vi "CTRE_Phoenix_PigeonIMU_HasResetOccurred.vi"(8 "error in":errorcluster, 11 "CTRE_PigeonIMU_DeviceRef":T1={"DeviceStatus"={"status"=FALSE, "code"=0, "source"=""}, "Device Number"=0, "Type"=352321536, "Device ID"=0, "Handle"=0, "UsageFrame"=0, "Library Path"=path ""} {"Type" items=["CAN"=352321536, "TalonSRX"=33554432]}) -> (0 "error out":errorcluster, 2 "Has Reset Occurred?":bool, 3 "CTRE_PigeonIMU_DeviceRef":T1={"DeviceStatus"={"status"=FALSE, "code"=0, "source"=""}, "Device Number"=0, "Type"=352321536, "Device ID"=0, "Handle"=0, "UsageFrame"=0, "Library Path"=path ""} {"Type" items=["CAN"=352321536, "TalonSRX"=33554432]})   [LabVIEW 2020]
doc: "Returns if the device has had a reset occur."
uses:
  <vilib>/Rock Robotics/WPI/ThirdParty/Phoenix-LabVIEW/Pigeon IMU/CTRE_PigeonIMU_DeviceRef.ctl
  <vilib>/Rock Robotics/WPI/ThirdParty/Phoenix-LabVIEW/Pigeon IMU/CTRE_PigeonIMU_ConnectionType.ctl
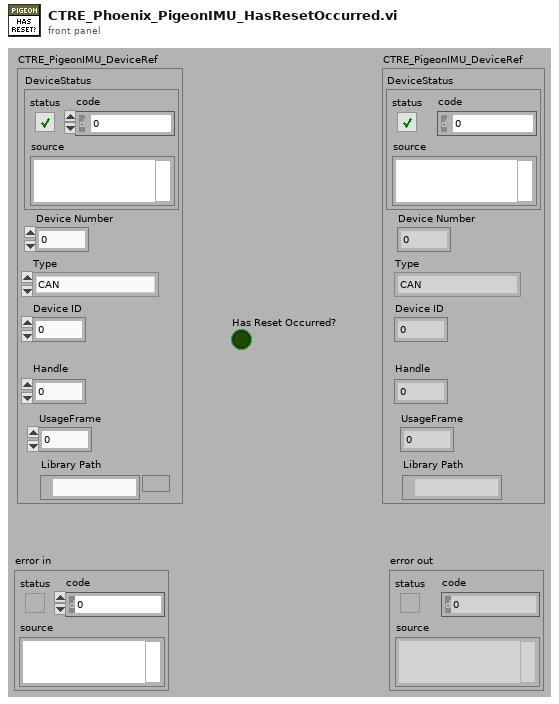
[diagram p1: front panel]
types:
  T1 = typedef "CTRE_PigeonIMU_DeviceRef.ctl" = cluster{"DeviceStatus":errorcluster, "Device Number":u8, "Type":T2, "Device ID":u32, "Handle":u64, "UsageFrame":u32, "Library Path":path}
  T2 = typedef "CTRE_PigeonIMU_ConnectionType.ctl" = u32
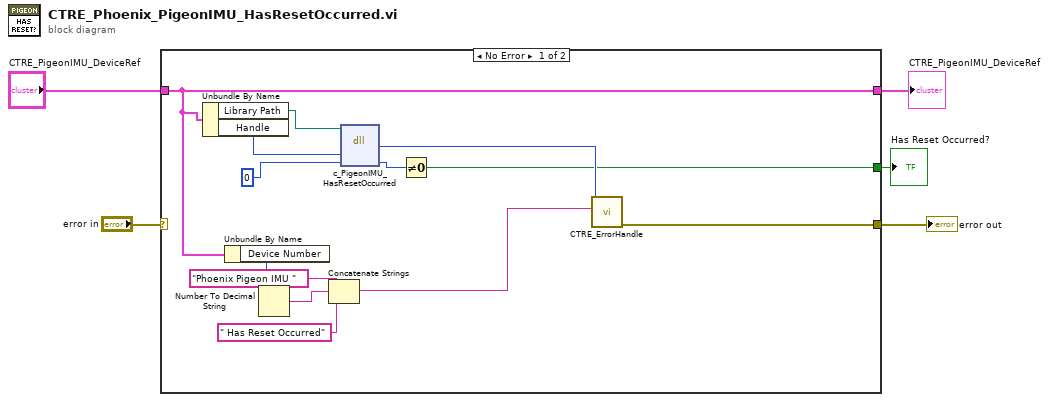
[diagram p0: block diagram]
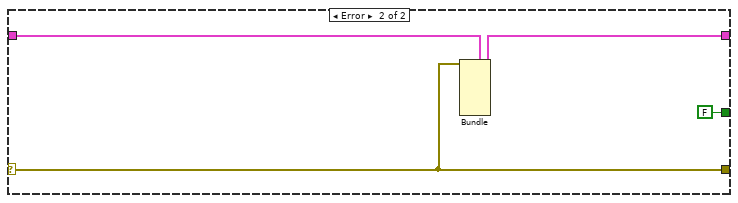
[diagram p2: hidden frame]
diagram:
  n1 = case shown="No Error" "error in" {
    selector: "error in" -> [_ w21]
    tunnel: "CTRE_PigeonIMU_DeviceRef" -> [w10 w22]
    tunnel: [w17 w21] -> w5
    tunnel: [w10 w20] -> w2
    tunnel: [w6 FALSE] -> w1
    frame No Error {
      n2 = Unbundle By Name(w10) -> ("Library Path"=w9:path, "Handle"=w8:u64)
      n3 = Unbundle By Name(w10) -> ("Device Number"=w13:u8)
      n4 = Number To Decimal String(number=w13) -> (decimal integer string=w15:string)  [unwired: 1 in]
      n5 = Concatenate Strings("Phoenix Pigeon IMU " ("string"), w15, " Has Reset Occurred" ("string")) -> (w11:string)
      n6 = dll-call lib="?" fn="c_PigeonIMU_HasResetOccurred"(path in=w9, "handle"=w8, "hasResetOccurred"=u32 0 ("appliedThrottle")) -> ("return type"=w12:i32, "hasResetOccurred"=w7:u8)  [unwired: 3 in, 2 out]
      n7 = Not Equal To 0?(x=w7) -> (x != 0?=w6:bool)
      n8 = call <vilib>:"CTRE_ErrorHandle.vi"("origin"=w11, "code"=w12) -> ("error out"=w17:errorcluster)  [unwired: 9 in]
    }
    frame Error {
      n9 = Bundle(cluster=w22, "DeviceStatus"=w21) -> (w20:T1)  [unwired: 6 in]
    }
  }
  "error out" <- w5
  "CTRE_PigeonIMU_DeviceRef" <- w2
  "Has Reset Occurred?" <- w1
